vi "Tasks.vi"(8 "error in (no error)":errorcluster, 11 "Node in":refnum<class "Node.lvclass">) -> (0 "error out":errorcluster, 2 "Tasks":refnum<class "Task.lvclass">[](array[class]), 3 "Node out":refnum<class "Node.lvclass">)   [LabVIEW 2020, in "VolatusConfig.lvlib" / "Node.lvclass"]
uses:
  Node.lvclass
  C:/dev/lv20CE/relink/lv-volatus/VolatusConfig/VolatusConfigElement/VolatusConfigElement.lvclass
  Task/Task.lvclass
  Meta Type.ctl
  VolatusConfigElement/VolatusConfigElement.lvclass/VolatusConfigElement.ctl
  VolatusConfigElement/Element.vi
  lv-cdm/CDM-Config/Config Lookup/Match Meta.vi
  lv-cdm/CDM-Config/Config Element/Owner.vi
  lv-cdm/CDM-Config/Config Manager/Lookup Descendant.vi
  lv-cdm/CDM-Config/Config Filter/Config Lookup.lvclass
  Node.lvclass/Node.ctl
  VolatusConfig.lvlib
  VolatusConfigElement/VolatusConfigElement.lvclass
  C:/dev/lv20CE/relink/lv-volatus/VolatusConfig/Task/Task.lvclass
  C:/dev/lv20CE/relink/lv-volatus/VolatusConfig/Node/Node.lvclass
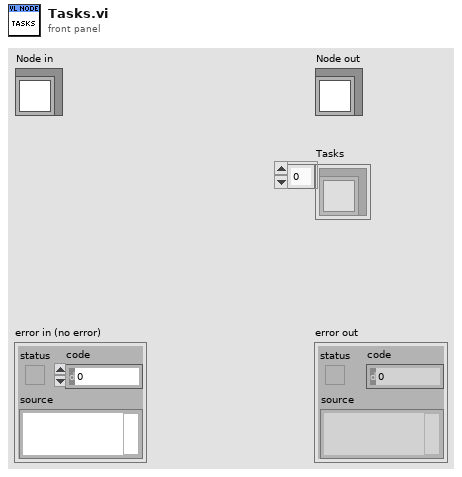
[diagram p1: front panel]
types:
  T1 = typedef "VolatusConfig.lvlib/Meta Type.ctl" = enum16{"UNKNOWN", "VL_System", "VL_Cluster", "VL_Node", "VL_Task", "VL_Group", "VL_Channel", "VL_Task_List", "VL_Scaling", "VL_Sensor", "VL_Sensor_List", "VL_Scale"}
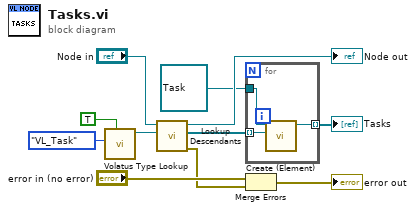
[diagram p0: block diagram]
diagram:
  n1 = call "Volatus Type Lookup.vi"("Don't Recurse Past Match (F)"=TRUE, "Meta Type"=Meta_Type."VL_Task") -> ("Config Lookup out"=w9:refnum<class "Config Lookup.lvclass">)  [unwired: 8 in, 1 out]
  n2 = call "Lookup Descendants.vi"("Lookup"=w9, "VolatusConfigElement in"="Node in") -> ("error out"=w5:errorcluster, "Descendants"=w8:refnum<class "Config Element.lvclass">[], "VolatusConfigElement out"=→"Node out":refnum<class "Node.lvclass">)  [unwired: 7 in]
  n3 = for {
    tunnel: w8 -> [w14] mode=indexing
    tunnel: [w13] -> w7 mode=indexing
    tunnel: refnum<class "Task.lvclass"> refnum ("VolatusConfig.lvlib:Task.lvclass") -> [w12]
    n4 = call "Create (Element).vi"("Element"=w14, "VolatusConfigElement in"=w12) -> ("VolatusConfigElement in"=w13:refnum<class "Task.lvclass">)  [unwired: 8 in, 1 out]
  }
  "Tasks" <- w7
  n5 = Merge Errors("error in (no error)", w5) -> (→"error out":errorcluster)
